vi "Pos. change(SubVI).vi"(7 "before pos":T1, 8 "Top":i32, 9 "Left":i32, 10 "Resize fl":bool) -> (0 "Resize fl 2":bool, 5 "after pos":T1)   [LabVIEW 2013]
uses:
  <vilib>/Utility/miscctls.llb/LVPositionTypeDef.ctl
panel:
  out "Position":T1
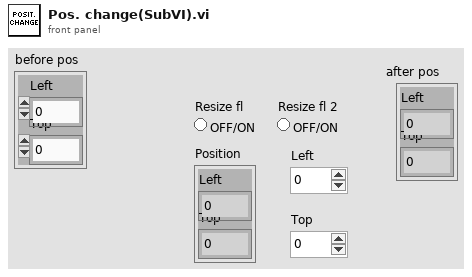
[diagram p1: front panel]
types:
  T1 = typedef "LVPositionTypeDef.ctl" = cluster{"Left":i32, "Top":i32}
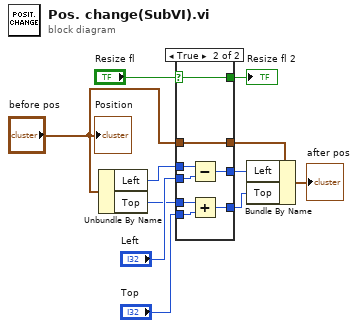
[diagram p0: block diagram]
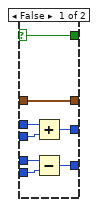
[diagram p2: hidden frame]
diagram:
  n1 = Unbundle By Name("before pos") -> ("Left"=w6:i32, "Top"=w5:i32)
  n2 = case shown="True" "Resize fl" {
    selector: "Resize fl" -> [w12 w20]
    tunnel: [w19 w27] -> w2
    tunnel: [w18 w26] -> w4
    tunnel: w6 -> [w17 w25]
    tunnel: w5 -> [w16 w24]
    tunnel: [w15 w23] -> w3
    tunnel: "before pos" -> [w15 w23]
    tunnel: "Left" -> [w14 w21]
    tunnel: "Top" -> [w13 w22]
    tunnel: [w12 w20] -> w1
    frame False {
      n3 = Add(x=w17, y=w14) -> (x+y=w18:i32)
      n4 = Subtract(x=w16, y=w13) -> (x-y=w19:i32)
    }
    frame True {
      n5 = Subtract(x=w25, y=w21) -> (x-y=w26:i32)
      n6 = Add(x=w24, y=w22) -> (x+y=w27:i32)
    }
  }
  "Resize fl 2" <- w1
  n7 = Bundle By Name(cluster=w3, "Left"=w4, "Top"=w2) -> (→"after pos":T1)
  "Position" <- "before pos"
